vi "lines_builder_novo.vi"(10 "Config data":path=path "C:/ATP/ATPDraw/Projects_Flavio/feeder123/config_novo.csv", 11 "Lines data":path=path "C:/ATP/ATPDraw/Projects_Flavio/feeder123/line data.csv") -> (0 "Outputs":string, 1 "To":dbl[](array[numeric]), 2 "From":dbl[](array[numeric]), 3 "Lines (out)":string)   [LabVIEW 2020]
uses:
  <vilib>/Utility/file.llb/Read Delimited Spreadsheet (DBL).vi
  <vilib>/Utility/file.llb/Read Delimited Spreadsheet (string).vi
panel:
  out "Array":bool[][](array[boolean])
  out "Numeric":dbl
  out "config":dbl[](array[numeric])
  out "Distance (miles)":dbl[](array[numeric])
  # "- Com lista de ouputs;\n-"
  # "LINES BUILDER"
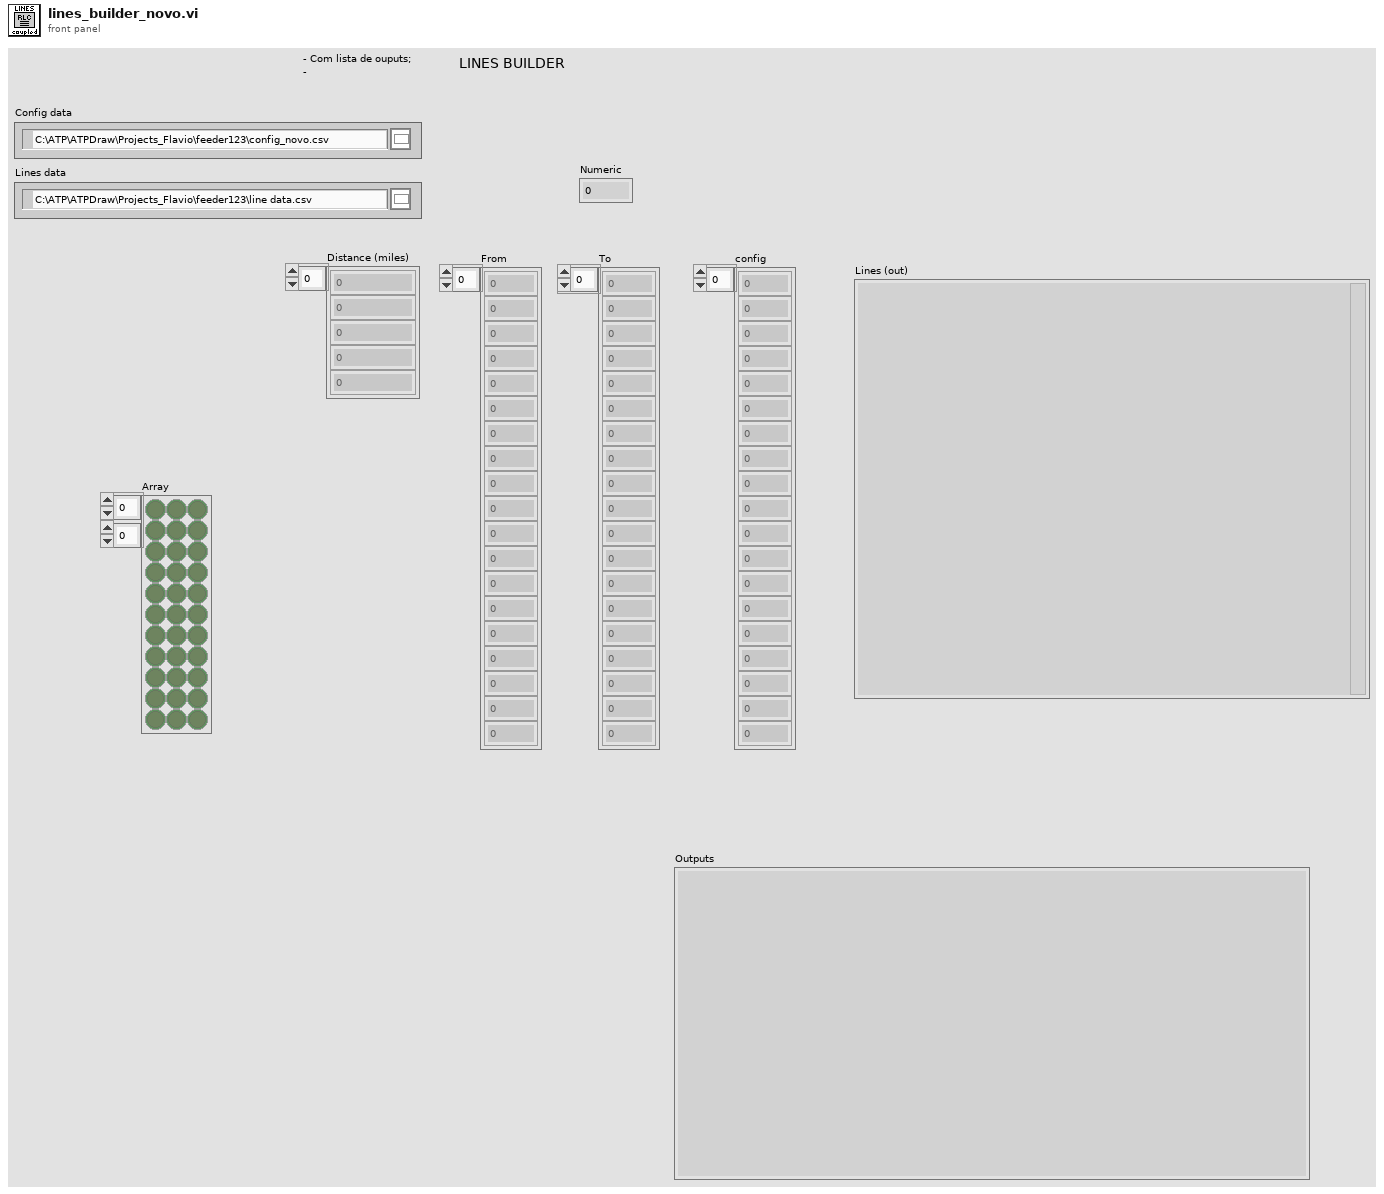
[diagram p1: front panel]
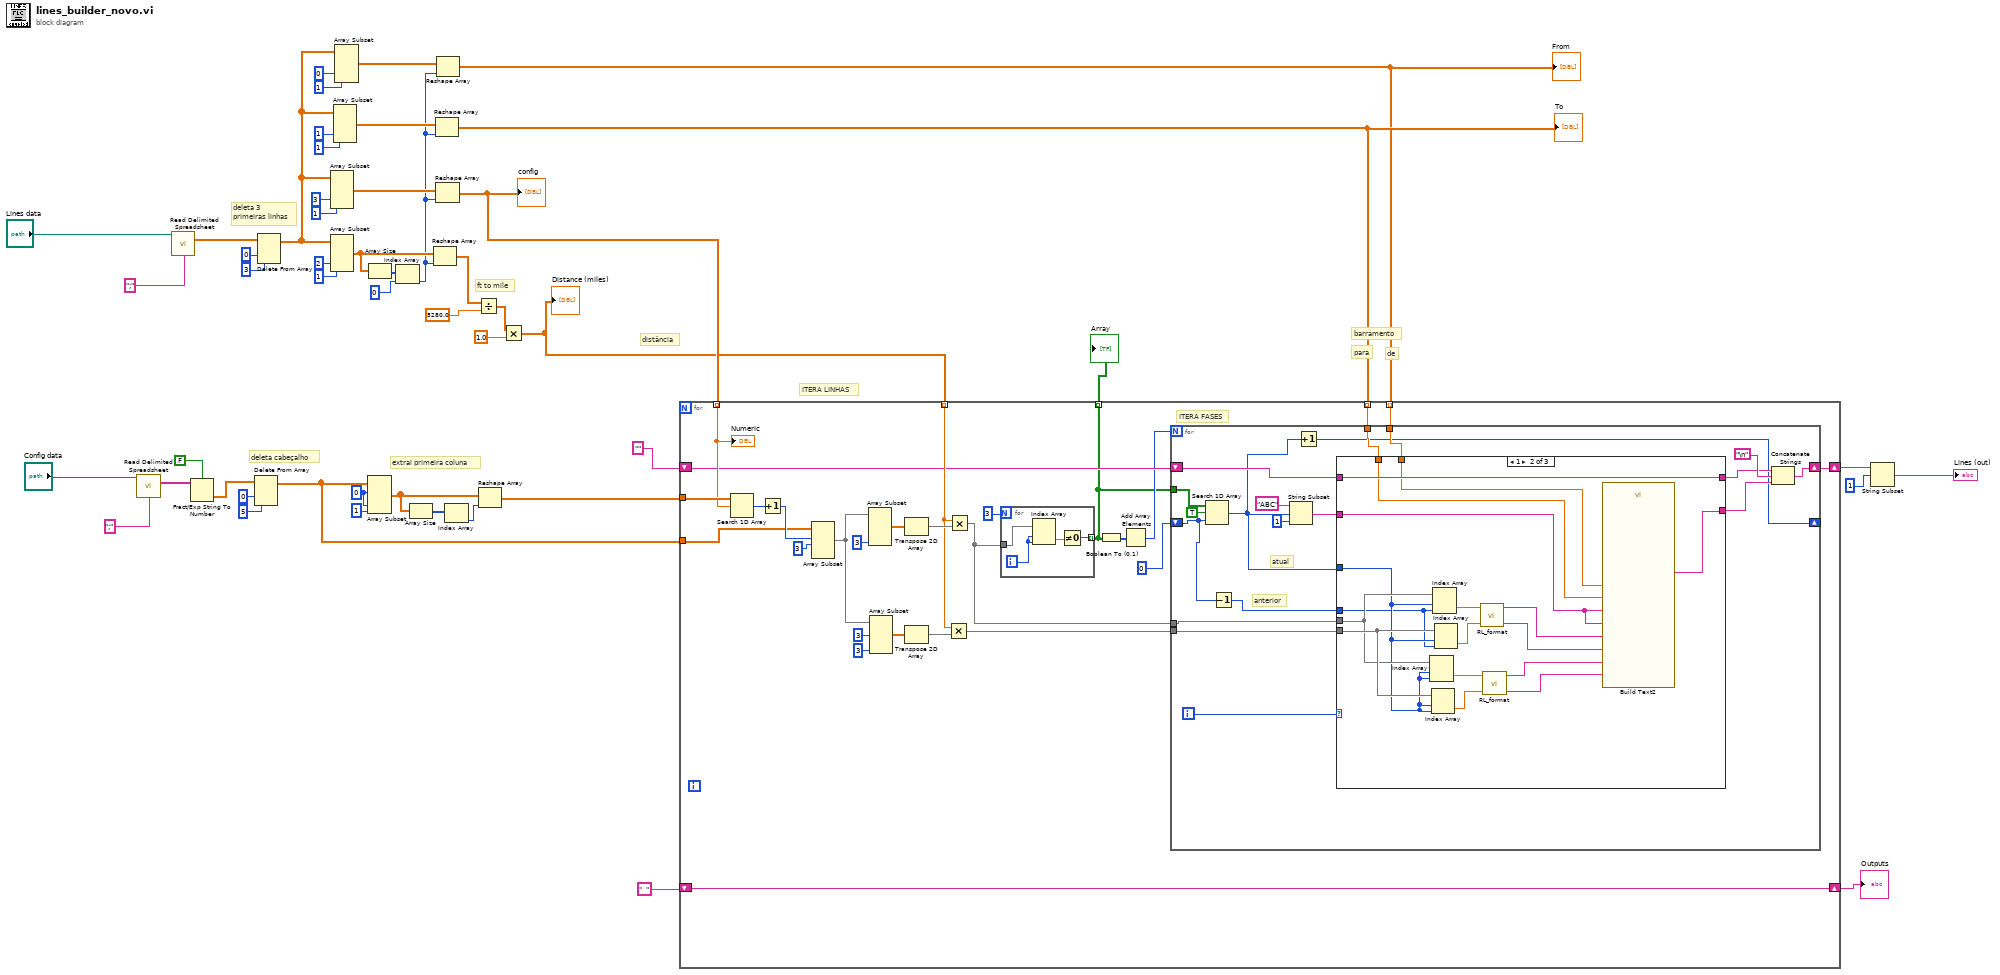
[diagram p0: block diagram]
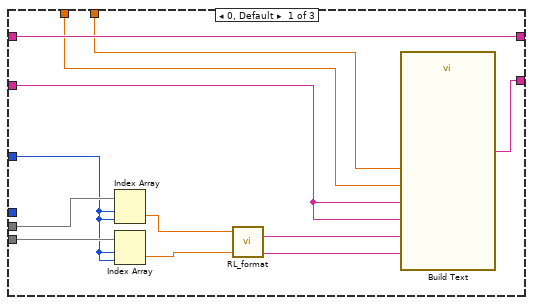
[diagram p2: hidden frame]
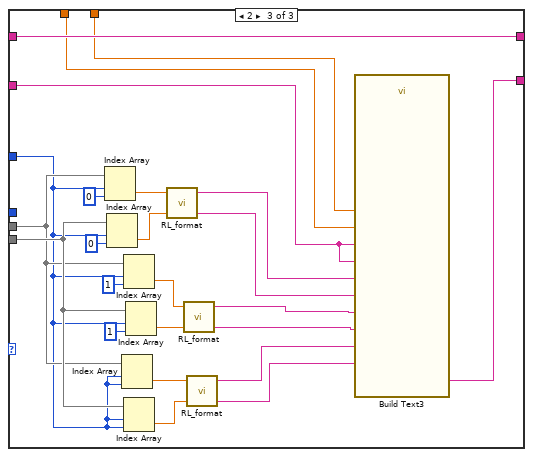
[diagram p3: hidden frame]
diagram:
  w11 = 0 ("index")
  # "ITERA LINHAS"
  # "extrai primeira coluna"
  # "deleta cabeçalho"
  # "barramento"
  # "para"
  # "de"
  # "distância"
  # "deleta 3\nprimeiras linhas"
  # "ft to mile"
  n1 = call-poly <vilib>:"Read Delimited Spreadsheet.vi"("file path (dialog if empty)"="Config data", "delimiter (\\t)"=";" ("delimiter (\\t)")) -> ("all rows"=w4:string[][])  [unwired: 8 in, 5 out]
  n2 = call-poly <vilib>:"Read Delimited Spreadsheet.vi"("file path (dialog if empty)"="Lines data", "delimiter (\\t)"=";" ("delimiter (\\t)")) -> ("all rows"=w19:dbl[][])  [unwired: 8 in, 5 out]
  n3 = Fract/Exp String To Number(use system decimal point (T)=FALSE, string=w4) -> (number=w3:dbl[][])  [unwired: 2 in, 1 out]
  n4 = Delete From Array(array=w3, length=5, index (row)=0) -> (array with subset deleted=w2:dbl[][])  [unwired: 1 in, 1 out]
  n5 = Delete From Array(array=w19, length=3, index (row)=0) -> (array with subset deleted=w36:dbl[][])  [unwired: 1 in, 1 out]
  n6 = Array Subset(array=w36, index (col)=3 ("index"), length (col)=1 ("length")) -> (w35:dbl[][])  [unwired: 2 in]
  n7 = Array Subset(array=w36, index (col)=2 ("index"), length (col)=1 ("length")) -> (w46:dbl[][])  [unwired: 2 in]
  n8 = Array Subset(array=w36, index (col)=1 ("index"), length (col)=1 ("length")) -> (w33:dbl[][])  [unwired: 2 in]
  n9 = Array Subset(array=w36, index (col)=0 ("index"), length (col)=1 ("length")) -> (w34:dbl[][])  [unwired: 2 in]
  n10 = Array Subset(array=w2, index (row)=w11, index (col)=w11, length (col)=1 ("length")) -> (w9:dbl[][])  [unwired: 1 in]
  n11 = Array Size(array=w46) -> (size(s)=w45:i32[])
  n12 = Index Array(array=w45, index=0) -> (element=w32:i32)
  n13 = Array Size(array=w9) -> (size(s)=w8:i32[])
  n14 = Reshape Array(w46, w32) -> (w14:dbl[])
  n15 = Reshape Array(w33, w32) -> (w29:dbl[])
  "To" <- w29
  n16 = Reshape Array(w35, w32) -> (w31:dbl[])
  "config" <- w31
  n17 = Reshape Array(w34, w32) -> (w28:dbl[])
  "From" <- w28
  n18 = Index Array(array=w8) -> (element=w7:i32)  [unwired: 1 in]
  n19 = Divide(x=w14, y=5280.0) -> (x/y=w12:dbl[])
  n20 = Reshape Array(w9, w7) -> (w6:dbl[])
  n21 = Multiply(x=w12, y=1.0) -> (x*y=w27:dbl[])
  "Distance (miles)" <- w27
  n22 = for {
    tunnel: w31 -> [w75] mode=indexing
    tunnel: w27 -> [w62] mode=indexing
    shift-right: [w61] -> w25
    shift-left: "" -> [w60]
    tunnel: w29 -> [w58] mode=indexing
    tunnel: w28 -> [w59] mode=indexing
    shift-right: [w77] -> w22
    shift-left: "  " -> [w77]
    tunnel: w6 -> [w76]
    tunnel: w2 -> [w71]
    tunnel: [w52] -> w1 mode=indexing
    # "ITERA FASES"
    n23 = Search 1D Array(1D array=w76, element=w75) -> (index of element=w74:i32)  [unwired: 1 in]
    n24 = Increment(x=w74) -> (x+1=w73:i32)
    n25 = Array Subset(array=w71, index (row)=w73, length (row)=3 ("length")) -> (w68:dbl[][])  [unwired: 2 in]
    n26 = Array Subset(array=w68, length (col)=3 ("length")) -> (w66:dbl[][])  [unwired: 3 in]
    n27 = Array Subset(array=w68, index (col)=3 ("index"), length (col)=3 ("length")) -> (w65:dbl[][])  [unwired: 2 in]
    n28 = Transpose 2D Array(2D array=w66) -> (transposed array=w64:dbl[][])
    n29 = Transpose 2D Array(2D array=w65) -> (transposed array=w63:dbl[][])
    n30 = Multiply(x=w62, y=w63) -> (x*y=w57:dbl[][])
    n31 = Multiply(x=w62, y=w64) -> (x*y=w55:dbl[][])
    n32 = for {
      N: 3 -> [_]
      tunnel: w55 -> [w80]
      tunnel: [w78] -> w52 mode=indexing
      i -> [w81]
      n33 = Index Array(array=w80, index (row)=w81, index (col)=w81) -> (element=w79:dbl)
      n34 = Not Equal To 0?(x=w79) -> (x != 0?=w78:bool)
    }
    n35 = Boolean To (0,1)(Boolean=w52) -> (0, 1=w53:i16[])
    n36 = Add Array Elements(numeric array=w53) -> (sum=w54:i16)
    n37 = for {
      N: w54 -> [_]
      tunnel: w55 -> [w94]
      shift-right: [w96] -> w61
      shift-left: w60 -> [w97]
      tunnel: w59 -> [w99]
      tunnel: w58 -> [w98]
      tunnel: w57 -> [w95]
      tunnel: w52 -> [w87]
      shift-right: [w84] -> _
      shift-left: 0 ("index of element") -> [w83]
      i -> [w100]
      # "anterior"
      # "atual"
      n38 = Search 1D Array(1D array=w87, element=TRUE, start index (0)=w83) -> (index of element=w85:i32)
      n39 = Decrement(x=w83) -> (x-1=w82:i32)
      n40 = String Subset(string="ABC", offset (0)=w85, length (rest)=1 ("length (rest)")) -> (substring=w88:string)
      n41 = Increment(x=w85) -> (x+1=w84:i32)
      n42 = case shown="1" w100 {
        tunnel: w99 -> [w110 w126 w146]
        tunnel: w98 -> [w102 w120 w138]
        tunnel: w97 -> [w111 w129 w153]
        tunnel: [w111 w129 w153] -> w92
        tunnel: [w112 w125 w139] -> w91
        tunnel: w95 -> [w108 w122 w143]
        tunnel: w94 -> [w109 w121 w142]
        tunnel: w85 -> [w105 w119 w135]
        tunnel: w88 -> [w101 w118 w134]
        tunnel: w82 -> [_ w115 _]
        frame 0, Default {
          n43 = Index Array(array=w109, index (row)=w105, index (col)=w105) -> (element=w107:dbl)
          n44 = Index Array(array=w108, index (row)=w105, index (col)=w105) -> (element=w106:dbl)
          n45 = call "RL_format.vi"("R"=w107, "X"=w106) -> ("R"=w103:string, "L"=w104:string)  [unwired: 6 in]
          n46 = call "Build Text"("fase_out"=w101, "L11"=w104, "node_in"=w110, "fase_in"=w101, "node_out"=w102, "R11"=w103) -> ("Result"=w112:string)  [unwired: 8 in, 1 out]
        }
        frame 1 {
          n47 = Index Array(array=w121, index (row)=w119, index (col)=w119) -> (element=w124:dbl)
          n48 = Index Array(array=w122, index (row)=w119, index (col)=w119) -> (element=w123:dbl)
          n49 = Index Array(array=w121, index (row)=w119, index (col)=w115) -> (element=w128:dbl)
          n50 = Index Array(array=w122, index (row)=w119, index (col)=w115) -> (element=w127:dbl)
          n51 = call "RL_format.vi"("R"=w128, "X"=w127) -> ("R"=w114:string, "L"=w113:string)  [unwired: 6 in]
          n52 = call "RL_format.vi"("R"=w124, "X"=w123) -> ("R"=w117:string, "L"=w116:string)  [unwired: 6 in]
          n53 = call "Build Text2"("fase_out"=w118, "L21"=w113, "L22"=w116, "node_in"=w126, "fase_in"=w118, "node_out"=w120, "R21"=w114, "R22"=w117) -> ("Result"=w125:string)  [unwired: 6 in, 1 out]
        }
        frame 2 {
          n54 = Index Array(array=w142, index (row)=w135, index (col)=0 ("disabled index (col)")) -> (element=w152:dbl)
          n55 = Index Array(array=w143, index (row)=w135, index (col)=0 ("disabled index (col)")) -> (element=w151:dbl)
          n56 = Index Array(array=w142, index (row)=w135, index (col)=w135) -> (element=w150:dbl)
          n57 = Index Array(array=w142, index (row)=w135, index (col)=1 ("disabled index (col)")) -> (element=w141:dbl)
          n58 = Index Array(array=w143, index (row)=w135, index (col)=w135) -> (element=w149:dbl)
          n59 = Index Array(array=w143, index (row)=w135, index (col)=1 ("disabled index (col)")) -> (element=w140:dbl)
          n60 = call "RL_format.vi"("R"=w152, "X"=w151) -> ("R"=w133:string, "L"=w132:string)  [unwired: 6 in]
          n61 = call "RL_format.vi"("R"=w141, "X"=w140) -> ("R"=w131:string, "L"=w130:string)  [unwired: 6 in]
          n62 = call "RL_format.vi"("R"=w150, "X"=w149) -> ("R"=w137:string, "L"=w136:string)  [unwired: 6 in]
          n63 = call "Build Text3"("node_in"=w146, "fase_in"=w134, "node_out"=w138, "fase_out"=w134, "R31"=w133, "L31"=w132, "R32"=w131, "L32"=w130, "R33"=w137, "L33"=w136) -> ("Result"=w139:string)  [unwired: 16 in, 1 out]
        }
      }
      n64 = Concatenate Strings(w92, "\n", w91) -> (w96:string)
    }
    "Numeric" <- w75
  }
  "Outputs" <- w22
  "Array" <- w1
  n65 = String Subset(string=w25, offset (0)=1) -> (substring=→"Lines (out)":string)  [unwired: 1 in]
